vi "Joystick Stiction Compensation.vi"(9 "A":dbl(slide) scale=0.0..1.0, 10 "B":dbl(slide) scale=0.0..1.0, 11 "Input":dbl(slide) scale=-1.0..1.0) -> (2 "Output":dbl)   [LabVIEW 2016]
uses:
  <vilib>/express/express arith-compare/Formula/XNode/ExpressFormulaBlockNode.xnode
panel:
  out "B":dbl
  out "A":dbl
  out "Input":dbl
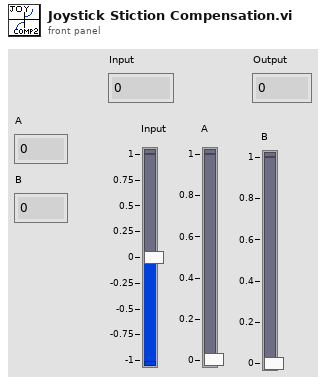
[diagram p1: front panel]
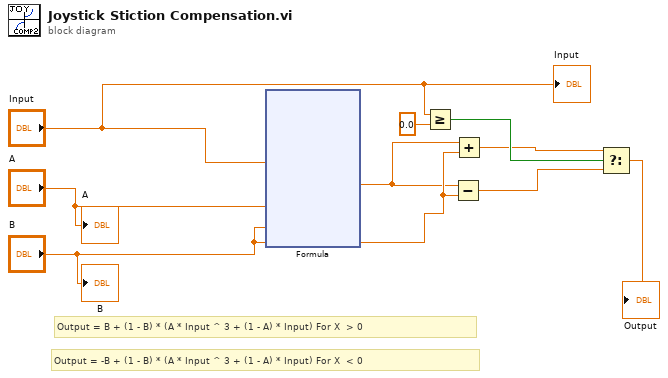
[diagram p0: block diagram]
diagram:
  # "Output = -B + (1 - B) * (A * Input ^ 3 + (1 - A) * Input) For X  < 0"
  # "Output = B + (1 - B) * (A * Input ^ 3 + (1 - A) * Input) For X  > 0"
  n1 = xnode "Formula"("Input"="Input", "A"="A", "B"="B") -> ("Result"=w2:dbl)  [unwired: 1 in, 1 out]
  n2 = Greater Or Equal?(x="Input", y=0.0) -> (x >= y?=w6:bool)
  n3 = Subtract(x=w2, y="B") -> (x-y=w3:dbl)
  n4 = Add(x=w2, y="B") -> (x+y=w5:dbl)
  n5 = Select(t=w5, s=w6, f=w3) -> (s? t:f=→"Output":dbl)
  "B" <- "B"
  "A" <- "A"
  "Input" <- "Input"
